vi "Set observer writing status.vi"(7 "writing":bool, 8 "error in (no error)":errorcluster, 10 "Message in":refnum<class "Message.lvclass">, 11 "Chat in":refnum<class "Chat.lvclass">) -> (0 "error out":errorcluster, 3 "Chat out":refnum<class "Chat.lvclass">)   [LabVIEW 2012, in "Chat.lvclass"]
uses:
  Chat.lvclass
  <vilib>/Distrio/Murmex/Message/Message.lvclass
  Chat.lvclass/Chat.ctl
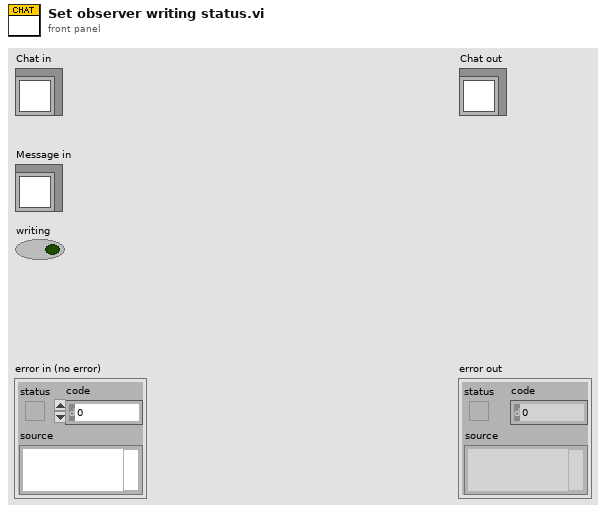
[diagram p1: front panel]
types:
  T1 = typedef "Chat.lvclass/observers_cluster.ctl" = cluster{"id":string, "writing":bool}
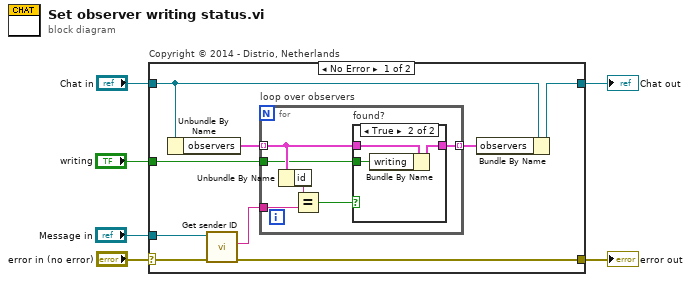
[diagram p0: block diagram]
diagram:
  n1 = case "Copyright © 2014 - Distrio, Netherlands" shown="No Error" "error in (no error)" {
    selector: "error in (no error)" -> [w15 w27]
    tunnel: [w14 w27] -> w3
    tunnel: [w10 w26] -> w2
    tunnel: "Chat in" -> [w11 w26]
    tunnel: "Message in" -> [w9 _]
    tunnel: "writing" -> [w8 _]
    frame No Error {
      n2 = Unbundle By Name(w11) -> ("observers"=w13:T1[])
      n3 = call <vilib>:"Get sender ID.vi"("error in (no error)"=w15, "Message in"=w9) -> ("error out"=w14:errorcluster, "sender"=w12:string)  [unwired: 7 in, 1 out]
      n4 = for "loop over observers" {
        tunnel: w13 -> [w19] mode=indexing
        tunnel: w12 -> [w20]
        tunnel: w8 -> [w18]
        tunnel: [w17] -> w7 mode=indexing
        n5 = Unbundle By Name(w19) -> ("id"=w21:string)
        n6 = Equal?(x=w21, y=w20) -> (x = y?=w16:bool)
        n7 = case "found?" shown="True" w16 {
          tunnel: w19 -> [w22 w25]
          tunnel: w18 -> [_ w24]
          tunnel: [w22 w23] -> w17
          frame False {
          }
          frame True {
            n8 = Bundle By Name(cluster=w25, "writing"=w24) -> (w23:T1)
          }
        }
      }
      n9 = Bundle By Name(cluster=w11, "observers"=w7) -> (w10:refnum<class "Chat.lvclass">)
    }
    frame Error {
    }
  }
  "error out" <- w3
  "Chat out" <- w2
